vi "Enqueue Sync Release.vi"(8 "error in (no error)":errorcluster, 11 "Instrument Owner in":refnum<class "Instrument Owner.lvclass">) -> (0 "error out":errorcluster, 3 "Instrument Owner out":refnum<class "Instrument Owner.lvclass">)   [LabVIEW 2020, in "Instrument Handler.lvlib" / "Instrument Owner.lvclass"]
doc: "Send a notification on the Enqueue Sync notifier to release the Instrument Owner."
uses:
  Instrument Owner.lvclass
  Instrument Owner.lvclass/Instrument Owner.ctl
  PPL/HDH.Data.Generic.lvlibp/Synchronization/Notifier/Notifier.lvclass
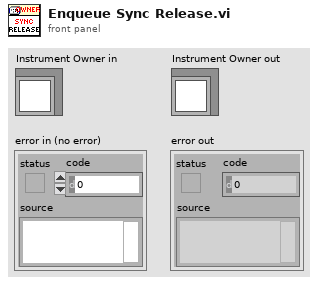
[diagram p1: front panel]
types:
  T1 = typedef "Instrument Handler.lvlib/Ctl_InstrumentSynchronicationCluster.ctl" = cluster{"Launched?":bool, "Driver Path":path, "Alias":string, "Connection Type":T2, "Pre Initialization Data":variant, "Enqueue Sync":refnum<class "Notifier.lvclass">, "Enqueue Lock":T3, "Owner Enqueuer":refnum<class "Message Enqueuer.lvclass">, "Owner":refnum<class "Sequencer Core.lvclass">, "Instrument ID":u32}
  T2 = typedef "HDH.Actor Framework.Core.Instrument Driver.lvlibp/Instrument Driver.lvclass/Ctl_ConnectionType.ctl" = enum16{"BuiltIn/System", "PXI/PCI", "USB", "GPIB", "VXI", "Serial", "TCP/IP", "cRIO", "SCXI", "cDAQ", "SwitchBlock", "SCC", "FireWire", "Accessory", "CAN", "SwitchBlock Device"}
  T3 = typedef "Semaphore RefNum" = refnum<k1>
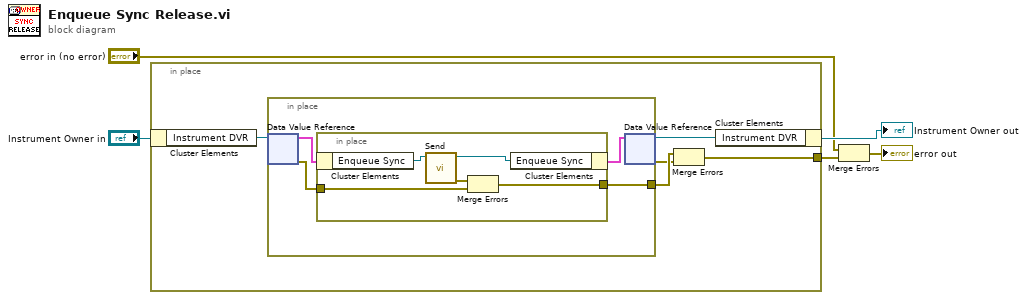
[diagram p0: block diagram]
diagram:
  n1 = in-place {
    in-place-border: [w7] -> w5
    n2 = in-place-cluster #1("Instrument Owner in") -> ("Instrument DVR"=w9:refnum<data-value>)
    n3 = in-place {
      in-place-border: [w14] -> w10
      n4 = in-place-dvr #2(w9) -> (w13:T1, w11:errorcluster)
      n5 = in-place {
        in-place-border: [w19] -> w14
        in-place-border: w11 -> [w18]
        n6 = in-place-cluster #3(w13) -> ("Enqueue Sync"=w16:refnum<class "Notifier.lvclass">)
        n7 = call "Send.vi"("Notifier in"=w16) -> ("error out"=w17:errorcluster, "Notifier out"=w15:refnum<class "Notifier.lvclass">)  [unwired: 9 in]
        n8 = Merge Errors(w17, w18) -> (w19:errorcluster)
        n9 = in-place-cluster #3("Enqueue Sync"=w15) -> (w12:T1)
      }
      n10 = in-place-dvr #2(w12) -> (w8:refnum<data-value>, w6:errorcluster)
    }
    n11 = Merge Errors(w10, w6) -> (w7:errorcluster)
    n12 = in-place-cluster #1("Instrument DVR"=w8) -> (→"Instrument Owner out":refnum<class "Instrument Owner.lvclass">)
  }
  n13 = Merge Errors("error in (no error)", w5) -> (→"error out":errorcluster)
